vi "SCLN_WaitInitReady.vi"(1 "error in (no error)":errorcluster) -> (0 "error out":errorcluster)   [LabVIEW 2015]
uses:
  SCLN_RW_Select.ctl
  SCLN_NOTIF_Select.ctl
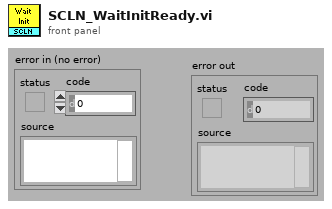
[diagram p1: front panel]
types:
  T1 = typedef "SCLN_NOTIF_Select.ctl" = enum16{"Server1", "Server2", "Server3", "Server4", "Server5", "Server6", "Server7", "Client1", "Client2", "Client3", "Client4", "Client5", "Client6", "Client7", "Client8", "Client9", "Client10", "Shutdown", "Init_Ready"}
  T2 = typedef "SCLN_RW_Select.ctl" = enum16{"Read", "Write"}
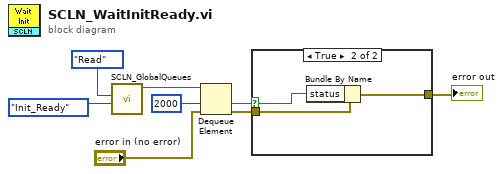
[diagram p0: block diagram]
diagram:
  n1 = call "SCLN_GlobalQueues.vi"("Element"=SCLN_NOTIF_Select."Init_Ready" ("Dome String Ctrl"), "Operation"=SCLN_RW_Select."Read" ("GBL_RW")) -> ("Read QueueID"=w5:refnum<queue>)  [unwired: 6 in, 1 out]
  n2 = Dequeue Element(queue=w5, timeout in ms (-1)=2000, error in (no error)="error in (no error)") -> (timed out?=w3:bool, error out=w2:errorcluster)  [unwired: 2 out]
  n3 = case shown="True" w3 {
    selector: w3 -> [_ w11]
    tunnel: w2 -> [w9 w12]
    tunnel: [w9 w10] -> w1
    frame False {
    }
    frame True {
      n4 = Bundle By Name(cluster=w12, "status"=w11) -> (w10:errorcluster)
    }
  }
  "error out" <- w1
